vi "scale8.vi"(9 "yDegree":dbl=10.0, 10 "xDegree":dbl=10.0, 11 "9dots":dbl[][](array[numeric])=[[-10.121699242325757, -7.417114276536165], [-0.2455631457321074, -8.018156632695227], [9.742835796667649, -7.770111532011539], [-10.34283427902477, -0.4009774143288431], [0.0, 0.0], [9.974111559079017, -0.1454241122747903], [-10.116610596371256, 7.666550305797061], [-0.15990313948414014, 7.866002027542072], [10.094520871915313, 7.895251816309939]]) -> (3 "ScaleArray":dbl[][](array[numeric]))   [LabVIEW 2011]
panel:
  out "x/y 2":dbl[](array[numeric])
  out "x/y":dbl[](array[numeric])
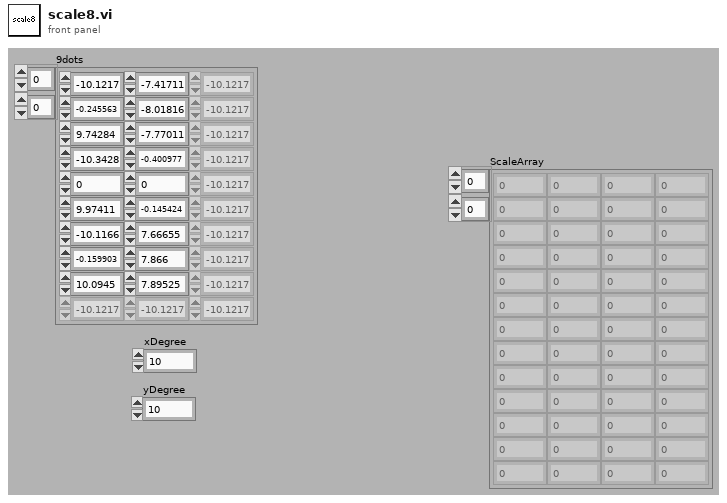
[diagram p1: front panel]
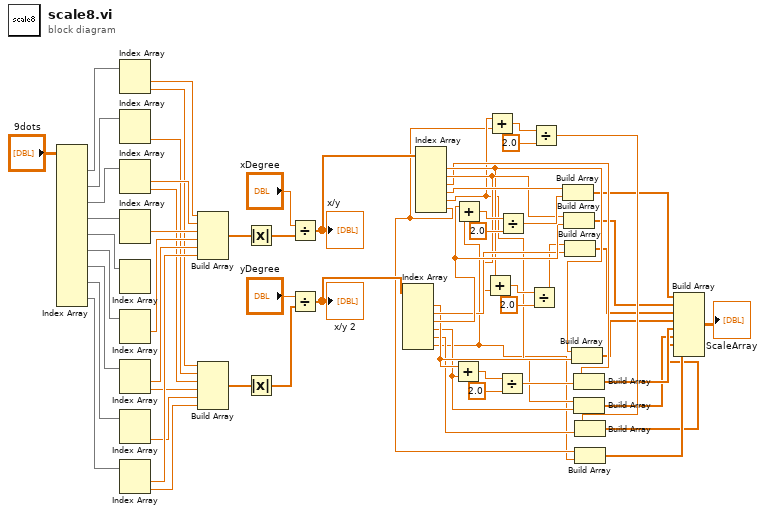
[diagram p0: block diagram]
diagram:
  n1 = Index Array(array="9dots") -> (element #1=w63:dbl[], element #2=w62:dbl[], element #3=w61:dbl[], element #4=w60:dbl[], element #5=w59:dbl[], element #6=w58:dbl[], element #7=w57:dbl[], element #8=w56:dbl[], element #9=w55:dbl[])  [unwired: 18 in]
  n2 = Index Array(array=w63) -> (element #1=w54:dbl, element #2=w48:dbl)  [unwired: 2 in]
  n3 = Index Array(array=w62) -> (element #2=w47:dbl)  [unwired: 2 in, 1 out]
  n4 = Index Array(array=w61) -> (element #1=w53:dbl, element #2=w46:dbl)  [unwired: 2 in]
  n5 = Index Array(array=w60) -> (element #1=w52:dbl)  [unwired: 2 in, 1 out]
  n6 = Index Array(array=w59) -> ()  [unwired: 2 in, 2 out]
  n7 = Index Array(array=w58) -> (element #1=w51:dbl)  [unwired: 2 in, 1 out]
  n8 = Index Array(array=w57) -> (element #1=w50:dbl, element #2=w45:dbl)  [unwired: 2 in]
  n9 = Index Array(array=w56) -> (element #2=w44:dbl)  [unwired: 2 in, 1 out]
  n10 = Index Array(array=w55) -> (element #1=w49:dbl, element #2=w43:dbl)  [unwired: 2 in]
  n11 = Build Array(w54, w53, w52, w51, w50, w49) -> (w38:dbl[])
  n12 = Build Array(w48, w47, w46, w45, w44, w43) -> (w40:dbl[])
  n13 = Absolute Value(x=w38) -> (abs(x)=w37:dbl[])
  n14 = Absolute Value(x=w40) -> (abs(x)=w39:dbl[])
  n15 = Divide(x="xDegree", y=w37) -> (x/y=w35:dbl[])
  "x/y" <- w35
  n16 = Divide(x="yDegree", y=w39) -> (x/y=w34:dbl[])
  "x/y 2" <- w34
  n17 = Index Array(array=w34) -> (element #1=w18:dbl, element #2=w28:dbl, element #3=w29:dbl, element #4=w17:dbl, element #5=w16:dbl, element #6=w10:dbl)  [unwired: 6 in]
  n18 = Index Array(array=w35) -> (element #1=w23:dbl, element #2=w25:dbl, element #3=w22:dbl, element #4=w33:dbl, element #5=w12:dbl, element #6=w11:dbl)  [unwired: 6 in]
  n19 = Add(x=w18, y=w17) -> (x+y=w20:dbl)
  n20 = Add(x=w29, y=w10) -> (x+y=w31:dbl)
  n21 = Add(x=w23, y=w25) -> (x+y=w26:dbl)
  n22 = Add(x=w12, y=w11) -> (x+y=w14:dbl)
  n23 = Divide(x=w20, y=2.0) -> (x/y=w19:dbl)
  n24 = Divide(x=w31, y=2.0) -> (x/y=w30:dbl)
  n25 = Divide(x=w26, y=2.0) -> (x/y=w24:dbl)
  n26 = Divide(x=w14, y=2.0) -> (x/y=w13:dbl)
  n27 = Build Array(w33, w30) -> (w9:dbl[])
  n28 = Build Array(w25, w29) -> (w8:dbl[])
  n29 = Build Array(w24, w28) -> (w7:dbl[])
  n30 = Build Array(w23, w18) -> (w6:dbl[])
  n31 = Build Array(w22, w19) -> (w5:dbl[])
  n32 = Build Array(w12, w17) -> (w4:dbl[])
  n33 = Build Array(w13, w16) -> (w1:dbl[])
  n34 = Build Array(w11, w10) -> (w2:dbl[])
  n35 = Build Array(w9, w8, w7, w6, w5, w4, w1, w2) -> (→"ScaleArray":dbl[][])
